vi "Producto.vi"(8 "error in (no error)":errorcluster, 9 "valor actual":u16, 10 "Item Names":string[][](array[string]), 11 "Bakery Actor in":refnum<class "Bakery Actor.lvclass">) -> (0 "error out":errorcluster, 3 "Bakery Actor out":refnum<class "Bakery Actor.lvclass">)   [LabVIEW 2019, in "Bakery Actor.lvlib" / "Bakery Actor.lvclass"]
uses:
  Bakery Actor.lvclass
  Bakery Actor.lvclass/Bakery Actor.ctl
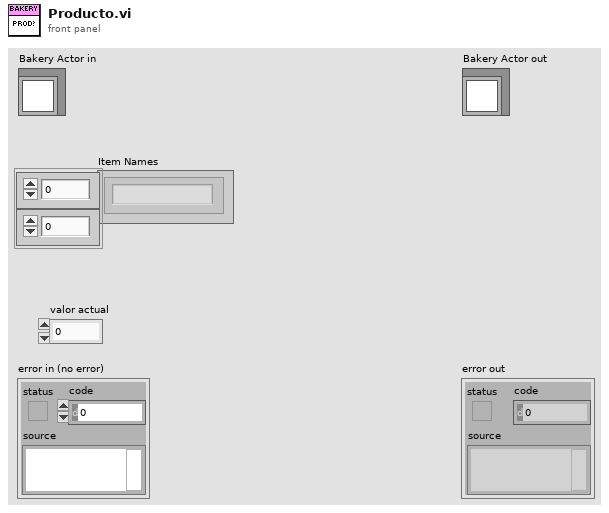
[diagram p1: front panel]
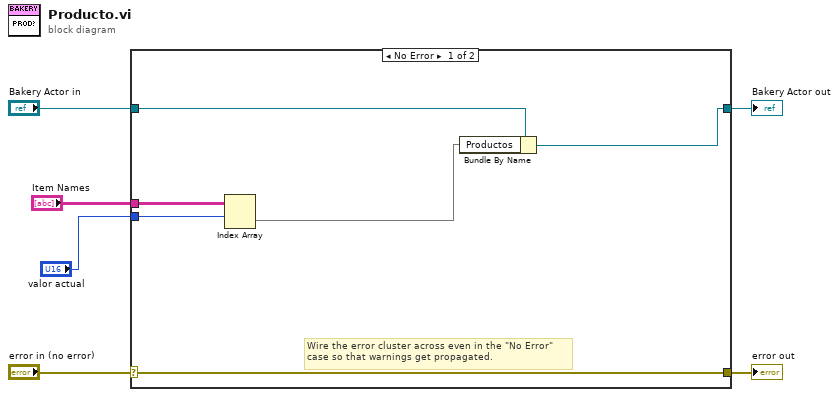
[diagram p0: block diagram]
diagram:
  n1 = case shown="No Error" "error in (no error)" {
    selector: "error in (no error)" -> [w12 w14]
    tunnel: [w12 w14] -> w5
    tunnel: [w9 w13] -> w3
    tunnel: "Bakery Actor in" -> [w10 w13]
    tunnel: "Item Names" -> [w8 _]
    tunnel: "valor actual" -> [w7 _]
    frame No Error {
      # "Wire the error cluster across even in the \"No Error\"\ncase so that warnings get propagated."
      n2 = Index Array(array=w8, index (row)=w7) -> (element=w11:string[])  [unwired: 1 in]
      n3 = Bundle By Name(cluster=w10, "Productos"=w11) -> (w9:refnum<class "Bakery Actor.lvclass">)
    }
    frame Error {
    }
  }
  "error out" <- w5
  "Bakery Actor out" <- w3
